vi "ST5 Save Act .vi"(4 "Unit Strings":string[](array[string]), 6 "Facteur Dir":bool, 7 "Units":u16, 8 "error in (no error)":errorcluster, 9 "Résolution Pas":dbl, 10 "Facteur Pas":dbl=1500.0, 11 "Actuator Settings":string) -> (0 "error out":errorcluster)   [LabVIEW 2019]
doc: "Use this template to build a VI to use as a subVI."
uses:
  <vilib>/Utility/config.llb/Write Key (Boolean).vi
  <vilib>/Utility/config.llb/Write Key (String).vi
  <vilib>/Utility/config.llb/Write Key (I32).vi
  <vilib>/Utility/config.llb/Write Key (Double).vi
  <vilib>/Utility/config.llb/NI_LVConfig.lvlib
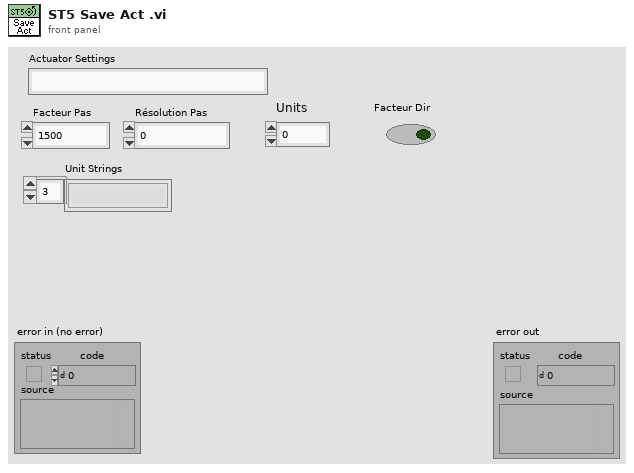
[diagram p1: front panel]
types:
  T1 = typedef "NI_LVConfig.lvlib/Config Data RefNum.ctl" = refnum<k1>
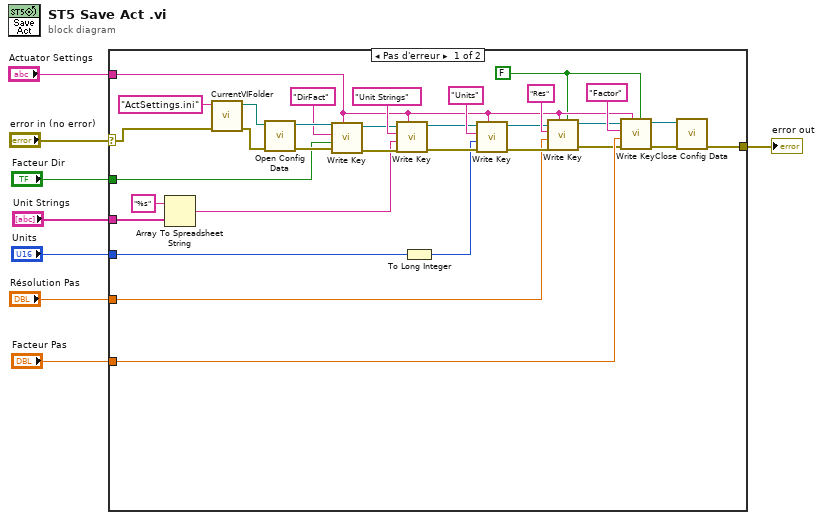
[diagram p0: block diagram]
diagram:
  n1 = case shown="Pas d'erreur" "error in (no error)" {
    selector: "error in (no error)" -> [w38 w41]
    tunnel: [w12 w41] -> w7
    tunnel: "Facteur Dir" -> [w33 _]
    tunnel: "Unit Strings" -> [w27 _]
    tunnel: "Units" -> [w24 _]
    tunnel: "Résolution Pas" -> [w18 _]
    tunnel: "Actuator Settings" -> [w10 _]
    tunnel: "Facteur Pas" -> [w16 _]
    frame No Error {
      w9 = FALSE ("use system decimal point (T)")
      n2 = Array To Spreadsheet String(array=w27, 3:"%s" ("format string")) -> (spreadsheet string=w25:string)  [unwired: 1 in]
      n3 = call <userlib>:"CurrentVIFolder.vi"("error in (no error)"=w38, "NomFichier"="ActSettings.ini") -> ("error out"=w37:errorcluster, "Chemin"=w40:path)  [unwired: 7 in, 1 out]
      n4 = call <vilib>:"Open Config Data.vi"("error in (no error)"=w37, "configuration file path"=w40) -> ("error out"=w34:errorcluster, "refnum"=w36:T1)  [unwired: 7 in, 1 out]
      n5 = call-poly <vilib>:"Write Key.vi"("section"=w10, "error in (no error)"=w34, "value"=w33, "key"="DirFact" ("section"), "refnum"=w36) -> ("error out"=w31:errorcluster, "refnum out"=w30:T1)  [unwired: 4 in, 1 out]
      n6 = call-poly <vilib>:"Write Key.vi"("section"=w10, "error in (no error)"=w31, "value"=w25, "key"="Unit Strings", "refnum"=w30) -> ("error out"=w29:errorcluster, "refnum out"=w23:T1)  [unwired: 4 in, 1 out]
      n7 = To Long Integer(number=w24) -> (32bit integer=w21:i32)
      n8 = call-poly <vilib>:"Write Key.vi"("section"=w10, "error in (no error)"=w29, "value"=w21, "key"="Units", "refnum"=w23) -> ("error out"=w20:errorcluster, "refnum out"=w19:T1)  [unwired: 4 in, 1 out]
      n9 = call-poly <vilib>:"Write Key.vi"("use system decimal point (T)"=w9, "section"=w10, "error in (no error)"=w20, "value"=w18, "key"="Res", "refnum"=w19) -> ("error out"=w15:errorcluster, "refnum out"=w14:T1)  [unwired: 3 in, 1 out]
      n10 = call-poly <vilib>:"Write Key.vi"("use system decimal point (T)"=w9, "section"=w10, "error in (no error)"=w15, "value"=w16, "key"="Factor", "refnum"=w14) -> ("error out"=w13:errorcluster, "refnum out"=w11:T1)  [unwired: 3 in, 1 out]
      n11 = call <vilib>:"Close Config Data.vi"("error in (no error)"=w13, "refnum"=w11) -> ("error out"=w12:errorcluster)  [unwired: 8 in, 1 out]
    }
    frame Error {
    }
  }
  "error out" <- w7
